vi "VALEW_ATC_Verify Non-concurrent.vi"(0 "GEA2 Reference In":refnum<k24>, 11 "Error In":errorcluster) -> (4 "GEA2 Reference Out":refnum<k24>, 6 "Pass/fail?":bool, 8 "Report Text":string, 15 "Error Out":errorcluster)   [LabVIEW 2016, in "Centauro.lvlib"]
doc: "This test covers the ATC algorithm when doing a non-concurrent fill. A non-concurrent fill does not allow both hot and cold valves to be on at the same time. The valves are operated in series, not in parallel."
uses:
  Projects/Centauro.lvlib
  Q:/Common/DLLs/GEA3/GeaCommunication.dll
  Common/DLLs/GEA3/GeaCommunication.dll
  Common/LabVIEW GEA2 Toolkit/LabVIEW_GEA2_Toolkit.lvlibp/type defs/Source_Destination.ctl
  Common/LabVIEW GEA2 Toolkit/LabVIEW_GEA2_Toolkit.lvlibp/type defs/ERD Write Data In.ctl
  Common/LabVIEW GEA2 Toolkit/LabVIEW_GEA2_Toolkit.lvlibp/type defs/Data Type.ctl
  Common/LabVIEW GEA2 Toolkit/LabVIEW_GEA2_Toolkit.lvlibp/type defs/ERD Read Data In.ctl
  Valew Common/type defs/MC_Cycle_Engine_Request_State.ctl
  <vilib>/DAQmx/write.llb/DAQmx Write (Analog DBL 1Chan 1Samp).vi
  <vilib>/DAQmx/create/channels.llb/DAQmx Create Channel (AO-Voltage-Basic).vi
  <vilib>/DAQmx/miscellaneous.llb/DAQmx Fill In Error Info.vi
  Common/LabVIEW GEA2 Toolkit/LabVIEW_GEA2_Toolkit.lvlibp
panel:
  out "Hot valve time (s) ATC 2":u16
  out "Cold valve time (s) ATC 2":u16
  out "Cold valve time (s) Calc 2":dbl
  out "Hot valve time (s) Calc 2":dbl
  out "High Times (s)":dbl[][](array[numeric])=[[0.048, 19.932000000000002, 0.0], [0.256, 9.626, 10.098], [0.254, 9.628, 10.098], [0.256, 9.625, 10.099], [0.047, 19.933, 0.0], [0.253, 10.701, 9.026], [0.255, 10.699, 9.026], [0.048, 19.932000000000002, 0.0], [0.258, 8.014, 11.708], [0.256, 8.016, 11.708], [0.256, 8.016, 11.708], [0.048, 19.932000000000002, 0.0], [0.254, 7.527, 12.199], [0.047, 19.933, 0.0], [0.253, 6.848, 12.879]]
  out "Hot inlet temp updated after 30sec?":bool
  out "Calc bath temp after seg gals":dbl
  out "Bath temp after seg gals":dbl
  out "Hot valve time (s) ATC":u16
  out "Cold valve time (s) ATC":u16
  out "Bath temp updated after segment fill?":bool
  out "Cold inlet temp updated after 30sec?":bool
  out "Cold valve pass?":bool
  out "Hot valve pass?":bool
  out "Cold valve time (s) Calc":dbl
  out "Hot valve time (s) Calc":dbl
  in  "Standalone?":bool
  # "Segment 1"
  # "Segment 2"
  # "off"
  # "on"
  # "off"
  # "on"
  # "off"
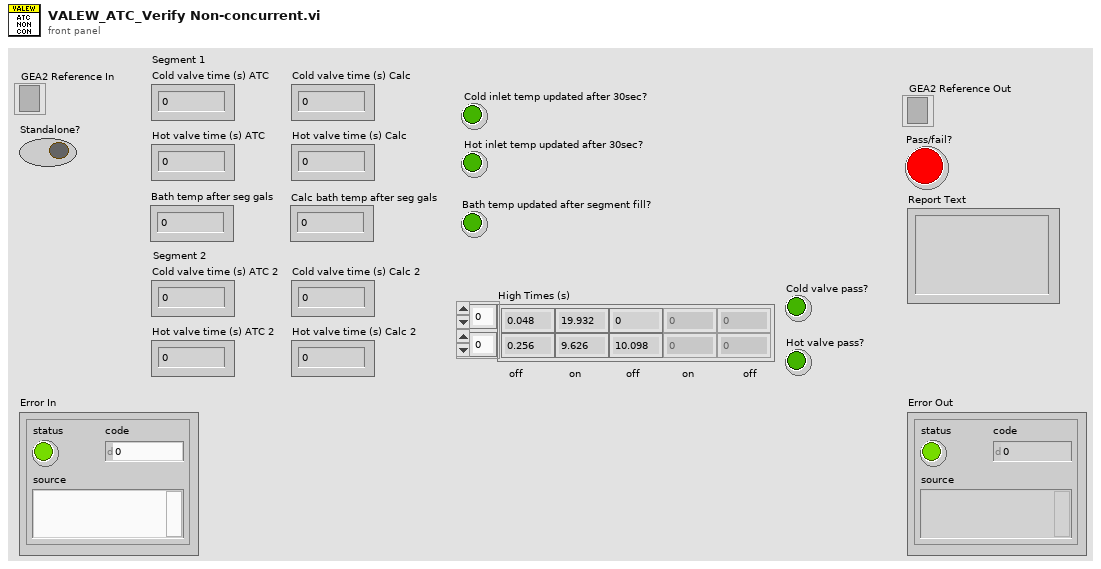
[diagram p1: front panel]
types:
  T1 = typedef "Centauro.lvlib/MC_Cycle_Engine_Request_State.ctl" = enum16{"Select", "Start", "Pause", "Resume", "Stop"}
  T2 = typedef "LabVIEW_GEA2_Toolkit.lvlibp/ERD Write Data In.ctl" = cluster{"ERD Number":u16, "Data Type":T3, "Data":string}
  T3 = typedef "LabVIEW_GEA2_Toolkit.lvlibp/Data Type.ctl" = enum16{"string", "boolean", "uint8_t", "uint16_t", "uint32_t", "uint64_t", "int8_t", "int16_t", "int32_t", "int64_t"}
  T4 = typedef "LabVIEW_GEA2_Toolkit.lvlibp/ERD Read Data In.ctl" = cluster{"ERD Number":u16, "Data Type":T3}
  T5 = enum16{"EQ (==)", "NE (!=)", "GT (>)", "LT (<)", "GE (>=)", "LE (<=)", "GTLT(> <)", "GELE (>= <=)", "GELT (>= <)", "GTLE (> <=)", "LTGT (< >)", "LEGE (<= >=)", "LEGT (<= >)", "LTGE (< >=)", "No Comparison"}
  T6 = typedef "LabVIEW_GEA2_Toolkit.lvlibp/Source_Destination.ctl" = cluster{"Source":u8, "Destination":u8}
  T7 = typedef "Centauro.lvlib/VALEW_ATC_Data.ctl" = cluster{"Accumulated hot gallons":dbl, "Accumulated cold gallons":dbl, "Current tub gallons":dbl, "Cold inlet temp (F)":dbl, "Hot inlet temp (F)":dbl, "Warm inlet temp (F)":dbl, "Hot valve time (s)":u16, "Cold valve time (s)":u16, "Current bath temp (F)":dbl, "Current water temp (F)":dbl, "Segment gallons":dbl}
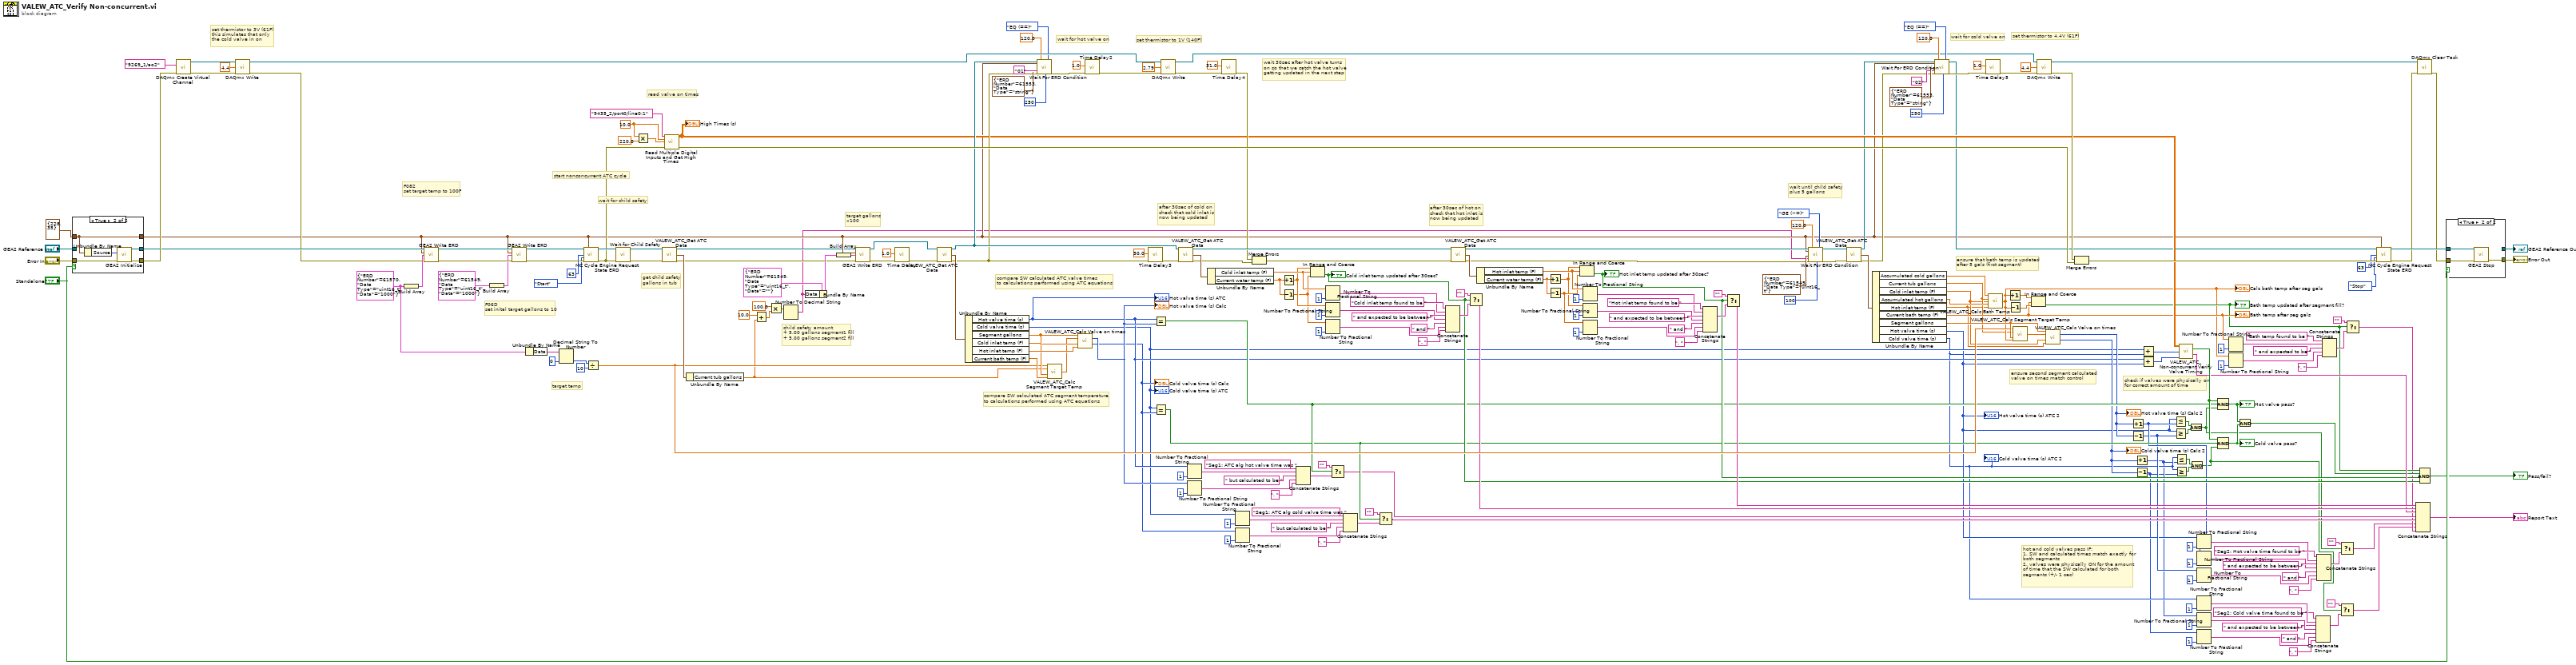
[diagram p0: block diagram]
diagram:
  w200 = 10.0 ("rate")
  w237 = T2 {"ERD Number"=61570, "Data Type"=enum."uint16_t", "Data"="1000"} ("ERD Write Data In")
  # "wait until child safety\nplus 5 gallons"
  # "hot and cold valves pass IF:\n1. SW and calculated times match exactly for\nboth segments\n2. valves were physically ON for the amount\nof time that the SW calculated for both\nsegments (+/- 1 sec)"
  # "compare SW calculated ATC valve times\nto calculations performed using ATC equations"
  # "compare SW calculated ATC segment temperature\nto calculations performed using ATC equations"
  # "wait 30sec after hot valve turns\non so that we catch the hot valve\ngetting updated in the next step"
  # "F06D\nset inital target gallons to 10"
  # "target gallons\nx100"
  # "check if valves were physically on\nfor correct amount of time"
  # "ensure second segment calculated\nvalve on times match control"
  # "ensure that bath temp is updated\nafter 5 gals (first segment)"
  # "wait for cold valve on"
  # "set thermistor to 4.4V (61F)"
  # "wait for hot valve on"
  # "set thermistor to 1V (140F)"
  # "after 30sec of hot on\ncheck that hot inlet is\nnow being updated"
  # "child safety amount\n+ 5.00 gallons segment1 fill\n+ 5.00 gallons segment2 fill"
  # "after 30sec of cold on\ncheck that cold inlet is\nnow being updated"
  # "get child safety\ngallons in tub"
  # "read valve on times"
  # "target temp"
  # "set thermistor to 3V (61F)\nthis simulates that only\nthe cold valve in on"
  # "wait for child safety"
  # "start nonconcurrent ATC cycle"
  # "F082\nset target temp to 100F"
  n1 = case shown="True" "Standalone?" {
    tunnel: T6 {"Source"=228, "Destination"=35} ("GEA Inputs") -> [w247 w250]
    tunnel: [w249 w253] -> w150
    tunnel: [w248 w252] -> w212
    tunnel: "Error In" -> [w248 w251]
    tunnel: "GEA2 Reference In" -> [w249 _]
    tunnel: [w247 w250] -> w9
    frame False {
    }
    frame True {
      n2 = Unbundle By Name(w250) -> ("Source"=w254:u8)
      n3 = call "GEA2 Initialize.vi"("Source Address"=w254, "error in"=w251) -> ("GEA2 Reference Out"=w253:refnum<k24>, "error out"=w252:errorcluster)  [unwired: 11 in, 1 out]
    }
  }
  n4 = call-poly <vilib>:"DAQmx Create Virtual Channel.vi"("physical channels"=tag "9269_1/ao2", "error in"=w212) -> ("task out"=w229:refnum<k21>, "error out"=w228:errorcluster)  [unwired: 12 in]
  n5 = call-poly <vilib>:"DAQmx Write.vi"("task/channels in"=w229, "data"=4.4, "error in"=w228) -> ("task out"=w197:refnum<k21>, "error out"=w149:errorcluster)  [unwired: 10 in, 1 out]
  n6 = Build Array(w237) -> (w236:T2[])
  n7 = call "GEA2 Write ERD.vi"("GEA2 Reference In"=w150, "GEA Inputs"=w9, "Write ERD List"=w236, "Error In"=w149) -> ("GEA2 Reference Out"=w225:refnum<k24>, "Error Out"=w224:errorcluster)  [unwired: 9 in, 1 out]
  n8 = Build Array(T2 {"ERD Number"=61549, "Data Type"=enum."uint16_t", "Data"="1000"} ("ERD Write Data In")) -> (w208:T2[])
  n9 = call "GEA2 Write ERD.vi"("GEA2 Reference In"=w225, "GEA Inputs"=w9, "Write ERD List"=w208, "Error In"=w224) -> ("GEA2 Reference Out"=w222:refnum<k24>, "Error Out"=w223:errorcluster)  [unwired: 9 in, 1 out]
  n10 = Unbundle By Name(w237) -> ("Data"=w235:string)
  n11 = Decimal String To Number(string=w235, default (0L)=u16 0 ("default (0 U32)")) -> (number=w233:u16)  [unwired: 1 in, 1 out]
  n12 = call "MC Cycle Engine Request State ERD.vi"("GEA2 Reference In"=w222, "GEA Inputs"=w9, "Cycle #"=u8 63, "MC Cycle Engine State"=MC_Cycle_Engine_Request_State."Start", "Error In"=w223) -> ("GEA2 Reference Out"=w242:refnum<k24>, "Error Out"=w161:errorcluster)  [unwired: 9 in]
  n13 = Divide(x=w233, y=u16 10) -> (x/y=w155:dbl)
  n14 = call "Wait for Child Safety.vi"("GEA2 Reference In"=w242, "Error In"=w161) -> ("GEA2 Reference Out"=w221:refnum<k24>, "Error Out"=w196:errorcluster)  [unwired: 9 in, 3 out]
  n15 = Multiply(x=w200, y=220.0) -> (x*y=w201:dbl)
  n16 = call "VALEW_ATC_Get ATC Data.vi"("GEA2 Reference In"=w221, "Error In"=w196) -> ("GEA2 Reference Out"=w4:refnum<k24>, "ATC Data"=w220:T7, "Error Out"=w7:errorcluster)  [unwired: 11 in]
  n17 = call "Read Multiple Digital Inputs and Get High Times.vi"("Lines"=tag "9435_2/port0/line0:1", "Rate (Hz)"=w200, "Samples"=w201, "Error In"=w161) -> ("High Times (s)"=w160:dbl[][], "Error Out"=w199:errorcluster)  [unwired: 10 in]
  "High Times (s)" <- w160
  n18 = Unbundle By Name(w220) -> ("Current tub gallons"=w8:dbl)
  n19 = Add(x=10.0, y=w8) -> (x+y=w11:dbl)
  n20 = Multiply(x=100.0, y=w11) -> (x*y=w12:dbl)
  n21 = Number To Decimal String(number=w12) -> (decimal integer string=w3:string)  [unwired: 1 in]
  n22 = Bundle By Name(cluster=T2 {"ERD Number"=61549, "Data Type"=enum."uint16_t", "Data"=""} ("ERD Write Data In"), "Data"=w3) -> (w13:T2)
  n23 = Build Array(w13) -> (w16:T2[])
  n24 = call "GEA2 Write ERD.vi"("GEA2 Reference In"=w4, "GEA Inputs"=w9, "Write ERD List"=w16, "Error In"=w7) -> ("GEA2 Reference Out"=w5:refnum<k24>, "Error Out"=w6:errorcluster)  [unwired: 9 in, 1 out]
  n25 = call "Time Delay"("error in (no error)"=w6, "Delay Time (s)"=1.0) -> ("error out"=w240:errorcluster)  [unwired: 9 in]
  n26 = call "VALEW_ATC_Get ATC Data.vi"("GEA2 Reference In"=w5, "Error In"=w240) -> ("GEA2 Reference Out"=w179:refnum<k24>, "ATC Data"=w239:T7, "Error Out"=w171:errorcluster)  [unwired: 11 in]
  n27 = Unbundle By Name(w239) -> ("Hot valve time (s)"=w31:u16, "Cold valve time (s)"=w29:u16, "Segment gallons"=w210:dbl, "Cold inlet temp (F)"=w218:dbl, "Hot inlet temp (F)"=w238:dbl, "Current bath temp (F)"=w209:dbl)
  "Cold valve time (s) ATC" <- w29
  "Hot valve time (s) ATC" <- w31
  n28 = call "Wait For ERD Condition.vi"("GEA2 Reference In"=w179, "GEA Inputs"=w9, "ERD Read Data"=T4 {"ERD Number"=61553, "Data Type"=enum."string"}, "Expected Low"="01", "Error In"=w171, "Timeout (s)"=120.0, "Loop Rate (ms)"=u32 250, "Comparison"=T5."EQ (==)") -> ("Error Out"=w168:errorcluster)  [unwired: 7 in, 4 out]
  n29 = call "VALEW_ATC_Calc Segment Target Temp.vi"("T(target)"=w155, "V(bath)"=w8, "V(segment)"=w210, "T(bath)"=w209) -> ("T(segment target)"=w211:dbl)  [unwired: 11 in]
  n30 = call "VALEW_ATC_Calc Valve on times.vi"("V(segment)"=w210, "T(segment target)"=w211, "T(cold inlet)"=w218, "T(hot inlet)"=w238) -> ("t(hot valve)"=w32:u16, "t(cold valve)"=w30:u16)  [unwired: 10 in]
  "Hot valve time (s) Calc" <- w32
  "Cold valve time (s) Calc" <- w30
  n31 = call "Time Delay2"("error in (no error)"=w168, "Delay Time (s)"=1.0) -> ("error out"=w169:errorcluster)  [unwired: 9 in]
  n32 = call "Time Delay3"("error in (no error)"=w171, "Delay Time (s)"=30.0) -> ("error out"=w194:errorcluster)  [unwired: 9 in]
  n33 = Equal?(x=w31, y=w32) -> (x = y?=w77:bool)
  n34 = Equal?(x=w29, y=w30) -> (x = y?=w76:bool)
  n35 = call-poly <vilib>:"DAQmx Write.vi"("task/channels in"=w197, "data"=2.79, "error in"=w169) -> ("task out"=w172:refnum<k21>, "error out"=w192:errorcluster)  [unwired: 10 in, 1 out]
  n36 = call "VALEW_ATC_Get ATC Data.vi"("GEA2 Reference In"=w179, "Error In"=w194) -> ("GEA2 Reference Out"=w189:refnum<k24>, "ATC Data"=w230:T7, "Error Out"=w186:errorcluster)  [unwired: 11 in]
  n37 = Number To Fractional String(number=w31, precision (6)=i16 1) -> (F-format string=w93:string)  [unwired: 2 in]
  n38 = Number To Fractional String(number=w32, precision (6)=i16 1) -> (F-format string=w91:string)  [unwired: 2 in]
  n39 = Unbundle By Name(w230) -> ("Cold inlet temp (F)"=w112:dbl, "Current water temp (F)"=w217:dbl)
  n40 = call "Time Delay4"("error in (no error)"=w192, "Delay Time (s)"=31.0) -> ("error out"=w164:errorcluster)  [unwired: 9 in]
  n41 = Number To Fractional String(number=w29, precision (6)=i16 1) -> (F-format string=w80:string)  [unwired: 2 in]
  n42 = Number To Fractional String(number=w30, precision (6)=i16 1) -> (F-format string=w82:string)  [unwired: 2 in]
  n43 = Merge Errors(w164, w186) -> (w187:errorcluster)
  n44 = Increment(x=w217) -> (x+1=w111:dbl)
  n45 = Decrement(x=w217) -> (x-1=w110:dbl)
  n46 = Concatenate Strings("Seg1: ATC alg hot valve time was ", w93, " but calculated to be ", w91, ". " ("string")) -> (w88:string)
  n47 = In Range and Coerce(upper limit=w111, x=w112, lower limit=w110) -> (In Range?=w97:bool)  [unwired: 1 out]
  "Cold inlet temp updated after 30sec?" <- w97
  n48 = Number To Fractional String(number=w112, precision (6)=i16 1) -> (F-format string=w116:string)  [unwired: 2 in]
  n49 = Number To Fractional String(number=w111, precision (6)=i16 1) -> (F-format string=w115:string)  [unwired: 2 in]
  n50 = Number To Fractional String(number=w110, precision (6)=i16 1) -> (F-format string=w134:string)  [unwired: 2 in]
  n51 = Select(t="", s=w77, f=w88) -> (s? t:f=w74:string)
  n52 = Concatenate Strings("Seg1: ATC alg cold valve time was ", w80, " but calculated to be ", w82, ". " ("string")) -> (w85:string)
  n53 = Select(t="", s=w76, f=w85) -> (s? t:f=w75:string)
  n54 = Concatenate Strings("Cold inlet temp found to be ", w116, " and expected to be between ", w115, " and " ("string"), w134, ". " ("string")) -> (w136:string)
  n55 = call "VALEW_ATC_Get ATC Data.vi"("GEA2 Reference In"=w189, "Error In"=w187) -> ("GEA2 Reference Out"=w62:refnum<k24>, "ATC Data"=w190:T7, "Error Out"=w61:errorcluster)  [unwired: 11 in]
  n56 = Select(t="", s=w97, f=w136) -> (s? t:f=w106:string)
  n57 = Unbundle By Name(w190) -> ("Hot inlet temp (F)"=w109:dbl, "Current water temp (F)"=w191:dbl)
  n58 = Increment(x=w191) -> (x+1=w107:dbl)
  n59 = Decrement(x=w191) -> (x-1=w108:dbl)
  n60 = In Range and Coerce(upper limit=w107, x=w109, lower limit=w108) -> (In Range?=w98:bool)  [unwired: 1 out]
  "Hot inlet temp updated after 30sec?" <- w98
  n61 = Number To Fractional String(number=w109, precision (6)=i16 1) -> (F-format string=w114:string)  [unwired: 2 in]
  n62 = Number To Fractional String(number=w107, precision (6)=i16 1) -> (F-format string=w113:string)  [unwired: 2 in]
  n63 = Number To Fractional String(number=w108, precision (6)=i16 1) -> (F-format string=w119:string)  [unwired: 2 in]
  n64 = Concatenate Strings("Hot inlet temp found to be ", w114, " and expected to be between ", w113, " and " ("string"), w119, ". " ("string")) -> (w117:string)
  n65 = Select(t="", s=w98, f=w117) -> (s? t:f=w105:string)
  n66 = call "Wait For ERD Condition.vi"("GEA2 Reference In"=w62, "GEA Inputs"=w9, "ERD Read Data"=T4 {"ERD Number"=61545, "Data Type"=enum."uint16_t"}, "Expected Low"=w3, "Error In"=w61, "Timeout (s)"=120.0, "Loop Rate (ms)"=u32 100, "Comparison"=T5."GE (>=)") -> ("GEA2 Reference Out"=w68:refnum<k24>, "Error Out"=w67:errorcluster)  [unwired: 7 in, 3 out]
  n67 = call "VALEW_ATC_Get ATC Data.vi"("GEA2 Reference In"=w68, "Error In"=w67) -> ("GEA2 Reference Out"=w154:refnum<k24>, "ATC Data"=w219:T7, "Error Out"=w152:errorcluster)  [unwired: 11 in]
  n68 = Unbundle By Name(w219) -> ("Accumulated cold gallons"=w215:dbl, "Current tub gallons"=w65:dbl, "Cold inlet temp (F)"=w64:dbl, "Accumulated hot gallons"=w216:dbl, "Hot inlet temp (F)"=w63:dbl, "Current bath temp (F)"=w137:dbl, "Segment gallons"=w156:dbl, "Hot valve time (s)"=w24:u16, "Cold valve time (s)"=w19:u16)
  "Bath temp after seg gals" <- w137
  "Cold valve time (s) ATC 2" <- w19
  "Hot valve time (s) ATC 2" <- w24
  n69 = call "Wait For ERD Condition.vi"("GEA2 Reference In"=w154, "GEA Inputs"=w9, "ERD Read Data"=T4 {"ERD Number"=61553, "Data Type"=enum."string"}, "Expected Low"="02", "Error In"=w152, "Timeout (s)"=120.0, "Loop Rate (ms)"=u32 250, "Comparison"=T5."EQ (==)") -> ("GEA2 Reference Out"=w153:refnum<k24>, "Error Out"=w166:errorcluster)  [unwired: 7 in, 3 out]
  n70 = call "Time Delay5"("error in (no error)"=w166, "Delay Time (s)"=1.0) -> ("error out"=w165:errorcluster)  [unwired: 9 in]
  n71 = call "VALEW_ATC_Calc Bath Temp.vi"("V(bath cold)"=w215, "V(bath)"=w65, "T(cold inlet)"=w64, "V(bath hot)"=w216, "T(hot inlet)"=w63) -> ("T(bath)"=w66:dbl)  [unwired: 10 in]
  "Calc bath temp after seg gals" <- w66
  n72 = Increment(x=w66) -> (x+1=w213:dbl)
  n73 = Decrement(x=w66) -> (x-1=w214:dbl)
  n74 = call "VALEW_ATC_Calc Segment Target Temp.vi"("T(target)"=w155, "V(bath)"=w65, "V(segment)"=w156, "T(bath)"=w66) -> ("T(segment target)"=w157:dbl)  [unwired: 11 in]
  n75 = In Range and Coerce(upper limit=w213, x=w137, lower limit=w214) -> (In Range?=w102:bool)  [unwired: 1 out]
  "Bath temp updated after segment fill?" <- w102
  n76 = call-poly <vilib>:"DAQmx Write.vi"("task/channels in"=w172, "data"=4.4, "error in"=w165) -> ("task out"=w163:refnum<k21>, "error out"=w162:errorcluster)  [unwired: 10 in, 1 out]
  n77 = call "VALEW_ATC_Calc Valve on times.vi"("V(segment)"=w156, "T(segment target)"=w157, "T(cold inlet)"=w64, "T(hot inlet)"=w63) -> ("t(hot valve)"=w48:u16, "t(cold valve)"=w46:u16)  [unwired: 10 in]
  "Hot valve time (s) Calc 2" <- w48
  "Cold valve time (s) Calc 2" <- w46
  n78 = Merge Errors(w162, w199) -> (w203:errorcluster)
  n79 = Increment(x=w48) -> (x+1=w26:u16)
  n80 = Decrement(x=w48) -> (x-1=w25:u16)
  n81 = Increment(x=w46) -> (x+1=w18:u16)
  n82 = Decrement(x=w46) -> (x-1=w17:u16)
  n83 = Add(x=w29, y=w19) -> (x+y=w159:u16)
  n84 = Add(x=w31, y=w24) -> (x+y=w158:u16)
  n85 = Less Or Equal?(x=w24, y=w26) -> (x <= y?=w28:bool)
  n86 = Greater Or Equal?(x=w24, y=w25) -> (x >= y?=w27:bool)
  n87 = Less Or Equal?(x=w19, y=w18) -> (x <= y?=w21:bool)
  n88 = Greater Or Equal?(x=w19, y=w17) -> (x >= y?=w22:bool)
  n89 = call "VALEW_ATC_Non-concurrent Verify Valve Timing.vi"("High Times (s)"=w160, "Total cold ON time (s)"=w159, "Total hot ON time (s)"=w158) -> ("Pass/Fail?"=w151:bool, "Report Text"=w104:string)  [unwired: 11 in]
  n90 = And(x=w28, y=w27) -> (x .and. y?=w23:bool)
  n91 = And(x=w21, y=w22) -> (x .and. y?=w20:bool)
  n92 = Number To Fractional String(number=w19, precision (6)=i16 1) -> (F-format string=w44:string)  [unwired: 2 in]
  n93 = Number To Fractional String(number=w18, precision (6)=i16 1) -> (F-format string=w45:string)  [unwired: 2 in]
  n94 = Number To Fractional String(number=w17, precision (6)=i16 1) -> (F-format string=w36:string)  [unwired: 2 in]
  n95 = Number To Fractional String(number=w24, precision (6)=i16 1) -> (F-format string=w50:string)  [unwired: 2 in]
  n96 = Number To Fractional String(number=w26, precision (6)=i16 1) -> (F-format string=w49:string)  [unwired: 2 in]
  n97 = Number To Fractional String(number=w25, precision (6)=i16 1) -> (F-format string=w58:string)  [unwired: 2 in]
  n98 = Compound Arithmetic op=AND(w151, w77, w23) -> (w101:bool)
  "Hot valve pass?" <- w101
  n99 = Compound Arithmetic op=AND(w151, w76, w20) -> (w100:bool)
  "Cold valve pass?" <- w100
  n100 = Number To Fractional String(number=w137, precision (6)=i16 1) -> (F-format string=w142:string)  [unwired: 2 in]
  n101 = Number To Fractional String(number=w66, precision (6)=i16 1) -> (F-format string=w140:string)  [unwired: 2 in]
  n102 = And(x=w101, y=w100) -> (x .and. y?=w99:bool)
  n103 = Concatenate Strings("Seg2: Cold valve time found to be ", w44, " and expected to be between ", w45, " and " ("string"), w36, ". " ("string")) -> (w34:string)
  n104 = Concatenate Strings("Seg2: Hot valve time found to be ", w50, " and expected to be between ", w49, " and " ("string"), w58, ". " ("string")) -> (w60:string)
  n105 = Concatenate Strings("Bath temp found to be ", w142, " and expected to be ", w140, ". " ("string")) -> (w139:string)
  n106 = Select(t="", s=w20, f=w34) -> (s? t:f=w33:string)
  n107 = Select(t="", s=w23, f=w60) -> (s? t:f=w47:string)
  n108 = Select(t="", s=w102, f=w139) -> (s? t:f=w73:string)
  n109 = call "MC Cycle Engine Request State ERD.vi"("GEA2 Reference In"=w153, "GEA Inputs"=w9, "Cycle #"=u8 63, "MC Cycle Engine State"=MC_Cycle_Engine_Request_State."Stop", "Error In"=w203) -> ("GEA2 Reference Out"=w202:refnum<k24>, "Error Out"=w188:errorcluster)  [unwired: 9 in]
  n110 = Concatenate Strings(w105, w106, w104, w74, w75, w47, w33, w73) -> (→"Report Text":string)
  n111 = call <vilib>:"DAQmx Clear Task.vi"("task in"=w163, "error in"=w188) -> ("error out"=w147:errorcluster)  [unwired: 13 in]
  n112 = Compound Arithmetic op=AND(w102, w99, w98, w97) -> (→"Pass/fail?":bool)
  n113 = case shown="True" "Standalone?" {
    tunnel: w147 -> [w256 w259]
    tunnel: w202 -> [w255 w258]
    tunnel: [w256 w257] -> w205
    tunnel: [w255 _] -> w206
    frame False {
    }
    frame True {
      n114 = call "GEA2 Stop.vi"("GEA2 Reference In"=w258, "Error In"=w259) -> ("Error Out"=w257:errorcluster)  [unwired: 13 in]
    }
  }
  "GEA2 Reference Out" <- w206
  "Error Out" <- w205
